vi "FSM - template by thetic.vi"() -> (15 "error out":errorcluster)   [LabVIEW 2024]
doc: "FSM - Template\nDistributed by Thetic Engineering Ltd. as open-source sample code without guarantees or warranties"
panel:
  # "Input"
  # "Output"
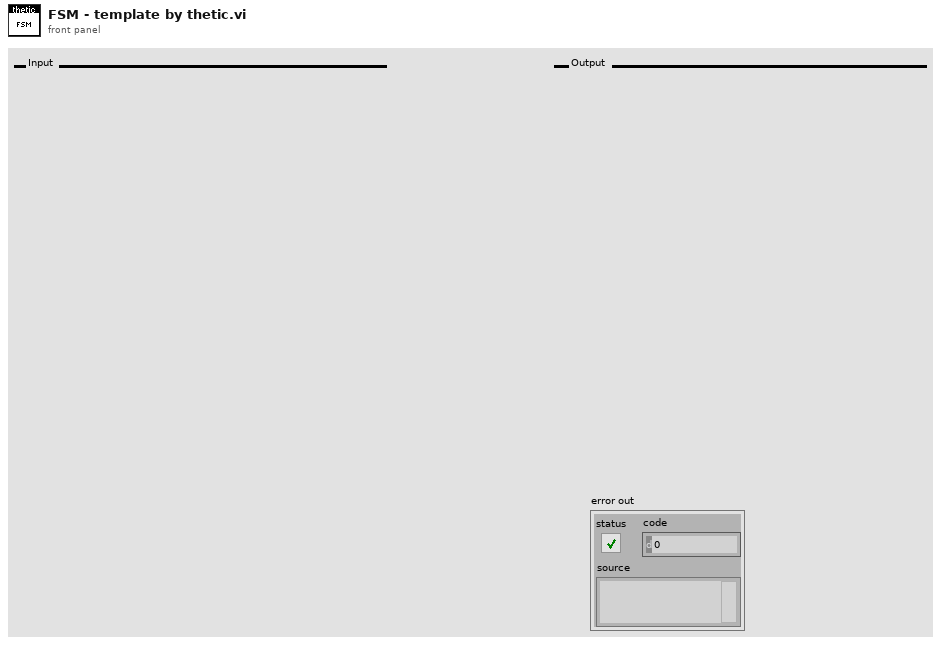
[diagram p1: front panel]
types:
  T1 = cluster{"numeric":i32, "string":string, "boolean":bool}
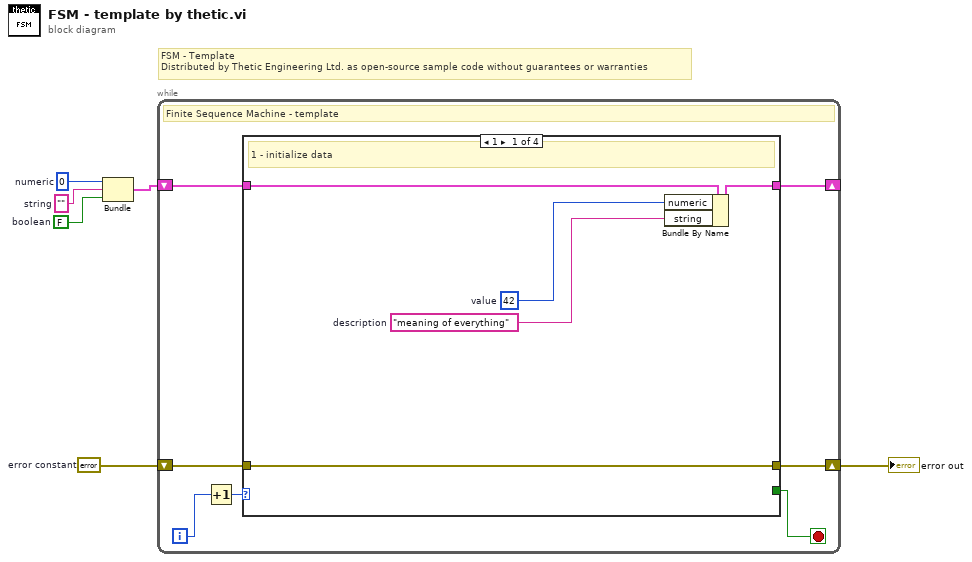
[diagram p0: block diagram]
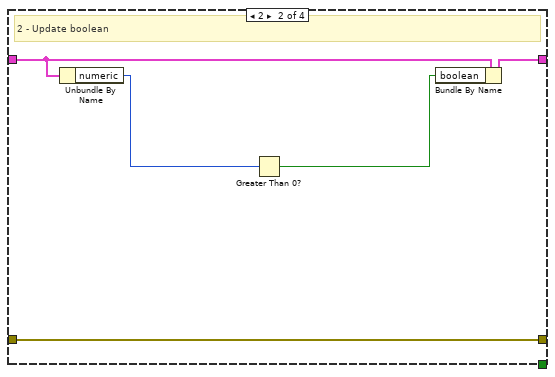
[diagram p2: hidden frame]
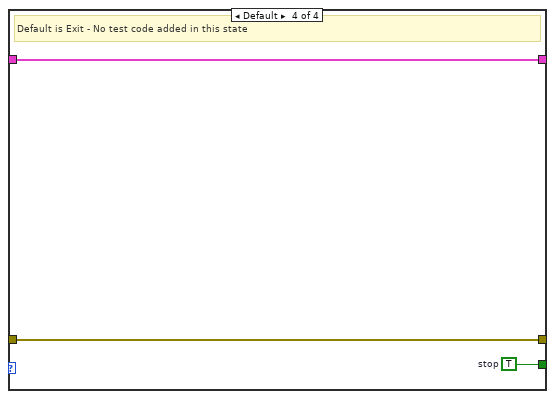
[diagram p4: hidden frame]
diagram:
  w1 = FALSE  # boolean
  w2 = ""  # string
  w3 = 0  # numeric
  w6 = errorcluster {"status"=FALSE, "code"=0, "source"=""}  # error constant
  # "FSM - Template\nDistributed by Thetic Engineering Ltd. as open-source sample code without guarantees or warranties"
  n1 = Bundle("numeric"=w3, "string"=w2, "boolean"=w1) -> (w4:T1)  [unwired: 1 in]
  n2 = while {
    shift-right: [w9] -> w5
    shift-left: w6 -> [w10]
    shift-right: [w8] -> _
    shift-left: w4 -> [w7]
    i -> [w12]
    stop <- w11 stop-if-true
    # "Finite Sequence Machine - template"
    n3 = Increment(x=w12) -> (x+1=w13:i32)
    n4 = case shown="1" w13 {
      tunnel: [_ _ _ w28] -> w11
      tunnel: w10 -> [w18 w23 w25 w27]
      tunnel: [w18 w23 w25 w27] -> w9
      tunnel: [w16 w22 w24 w26] -> w8
      tunnel: w7 -> [w17 w21 w24 w26]
      frame 1 {
        w14 = "meaning of everything"  # description
        w15 = 42  # value
        # "1 - initialize data"
        n5 = Bundle By Name(cluster=w17, "numeric"=w15, "string"=w14) -> (w16:T1)
      }
      frame 2 {
        # "2 - Update boolean"
        n6 = Unbundle By Name(w21) -> ("numeric"=w20:i32)
        n7 = Greater Than 0?(x=w20) -> (x > 0?=w19:bool)
        n8 = Bundle By Name(cluster=w21, "boolean"=w19) -> (w22:T1)
      }
      frame 3 {
        # "3 - Cleanup"
      }
      frame Default {
        w28 = TRUE  # stop
        # "Default is Exit - No test code added in this state"
      }
    }
  }
  "error out" <- w5
